vi "Post-Install Custom Action.vi"(10 "Variant":variant) -> (0 "error out":errorcluster)   [LabVIEW 2017]
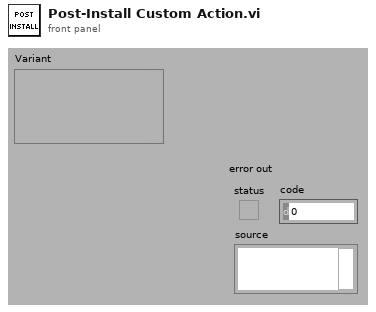
[diagram p1: front panel]
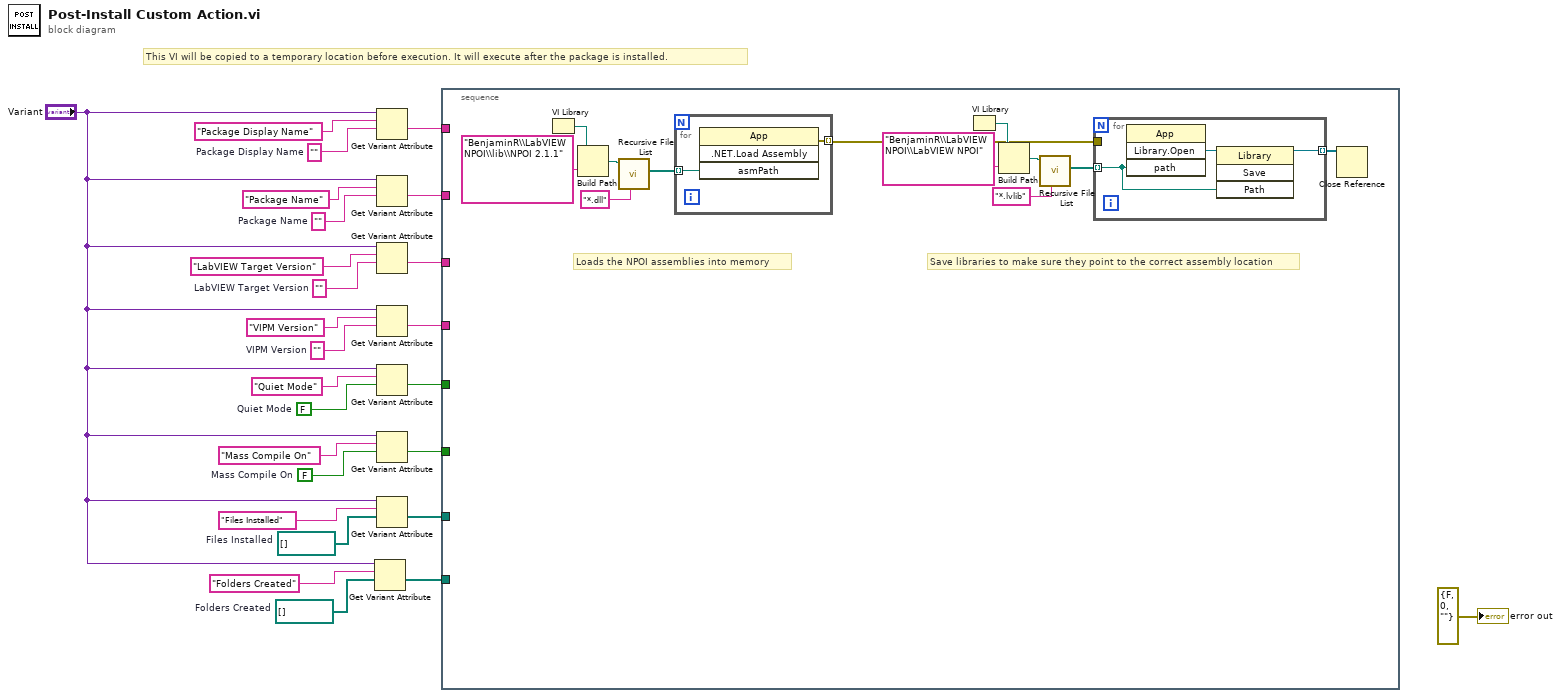
[diagram p0: block diagram]
diagram:
  w1 = path[] []  # Folders Created
  w2 = path[] []  # Files Installed
  w8 = FALSE  # Mass Compile On
  w9 = ""  # Package Display Name
  w16 = FALSE  # Quiet Mode
  w19 = ""  # VIPM Version
  w21 = ""  # LabVIEW Target Version
  w23 = ""  # Package Name
  # "This VI will be copied to a temporary location before execution. It will execute after the package is installed."
  n1 = Get Variant Attribute(Variant="Variant", name="Folders Created", default value (empty Variant)=w1) -> (value=w6:path[])  [unwired: 1 in, 3 out]
  n2 = Get Variant Attribute(Variant="Variant", name="Package Display Name", default value (empty Variant)=w9) -> (value=w15:string)  [unwired: 1 in, 3 out]
  n3 = Get Variant Attribute(Variant="Variant", name="Package Name", default value (empty Variant)=w23) -> (value=w14:string)  [unwired: 1 in, 3 out]
  n4 = Get Variant Attribute(Variant="Variant", name="LabVIEW Target Version", default value (empty Variant)=w21) -> (value=w13:string)  [unwired: 1 in, 3 out]
  n5 = Get Variant Attribute(Variant="Variant", name="VIPM Version", default value (empty Variant)=w19) -> (value=w12:string)  [unwired: 1 in, 3 out]
  n6 = Get Variant Attribute(Variant="Variant", name="Quiet Mode", default value (empty Variant)=w16) -> (value=w11:bool)  [unwired: 1 in, 3 out]
  n7 = Get Variant Attribute(Variant="Variant", name="Mass Compile On", default value (empty Variant)=w8) -> (value=w10:bool)  [unwired: 1 in, 3 out]
  n8 = Get Variant Attribute(Variant="Variant", name="Files Installed", default value (empty Variant)=w2) -> (value=w5:path[])  [unwired: 1 in, 3 out]
  n9 = stacked-sequence {
    tunnel: w15 -> [_]
    tunnel: w14 -> [_]
    tunnel: w13 -> [_]
    tunnel: w12 -> [_]
    tunnel: w11 -> [_]
    tunnel: w10 -> [_]
    tunnel: w5 -> [_]
    tunnel: w6 -> [_]
    frame #0 {
      # "Save libraries to make sure they point to the correct assembly location"
      # "Loads the NPOI assemblies into memory"
      n10 = VI Library() -> (path=w38:path)
      n11 = Build Path(base path=w38, name or relative path="BenjaminR\\LabVIEW NPOI\\lib\\NPOI 2.1.1") -> (appended path=w36:path)
      n12 = call <vilib>:"Recursive File List.vi"("pattern"="*.dll", "Folder Path"=w36) -> ("All Files in Dir"=w34:path[])  [unwired: 5 in, 4 out]
      n13 = for {
        tunnel: w34 -> [w43] mode=indexing
        tunnel: [w42] -> w27 mode=indexing
        n14 = invoke class="App" method=".NET.Load Assembly"("asmPath"=w43) -> (error out=w42:errorcluster)  [unwired: 3 in, 3 out]
      }
      n15 = VI Library() -> (path=w30:path)
      n16 = Build Path(base path=w30, name or relative path="BenjaminR\\LabVIEW NPOI\\LabVIEW NPOI") -> (appended path=w32:path)
      n17 = call <vilib>:"Recursive File List.vi"("pattern"="*.lvlib", "Folder Path"=w32) -> ("All Files in Dir"=w29:path[])  [unwired: 5 in, 4 out]
      n18 = for {
        tunnel: w29 -> [w40] mode=indexing
        tunnel: [w39] -> w28 mode=indexing
        tunnel: w27 -> [_]
        n19 = invoke class="App" method="Library.Open"("path"=w40) -> ("Open Library"=w41:refnum<vi>)  [unwired: 3 in, 3 out]
        n20 = invoke class="Library" method="Save"(reference=w41, "Path"=w40) -> (reference out=w39:refnum<vi>)  [unwired: 2 in, 3 out]
      }
      n21 = Close Reference(reference=w28) -> ()  [unwired: 1 in, 1 out]
    }
  }
  "error out" <- errorcluster {"status"=FALSE, "code"=0, "source"=""} ("error out")
